vi "GetSetterAccessorInfo.vi"(8 "error in (no error)":errorcluster, 11 "PropertyBinder in":refnum<class "PropertyBinder.lvclass">) -> (0 "error out":errorcluster, 2 "SetterAccessorInfo":T1[](array[typedef]), 3 "PropertyBinder out":refnum<class "PropertyBinder.lvclass">)   [LabVIEW 2023, in "PropertyBinder.lvclass"]
uses:
  PropertyBinder.lvclass
  PropertyBinder.lvclass/PropertyBinder.ctl
  ClassReflector/AccessorTypeEnum.ctl
  ClassReflector/ClassReflector.lvclass
  ClassReflector/AccessorInfoCluster.ctl
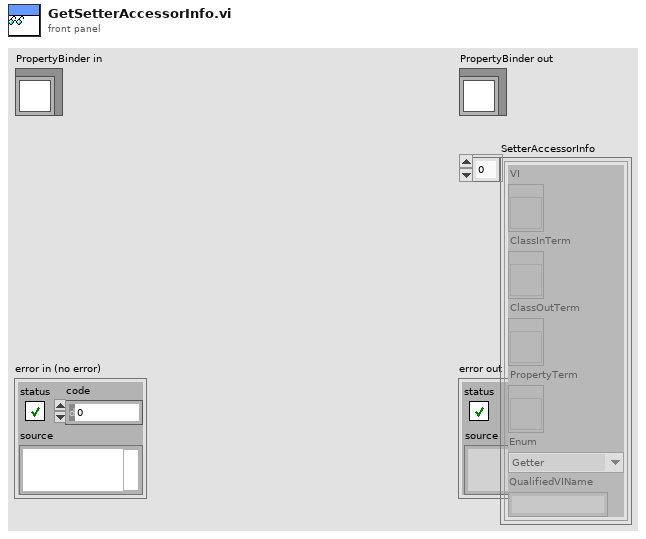
[diagram p1: front panel]
types:
  T1 = typedef "ClassReflector.lvclass/AccessorInfoCluster.ctl" = cluster{"VI":refnum<vi>, "ClassInTerm":refnum<vi>, "ClassOutTerm":refnum<vi>, "PropertyTerm":refnum<vi>, "Enum":T2, "QualifiedVIName":string}
  T2 = typedef "ClassReflector.lvclass/AccessorTypeEnum.ctl" = enum16{"Getter", "Setter"}
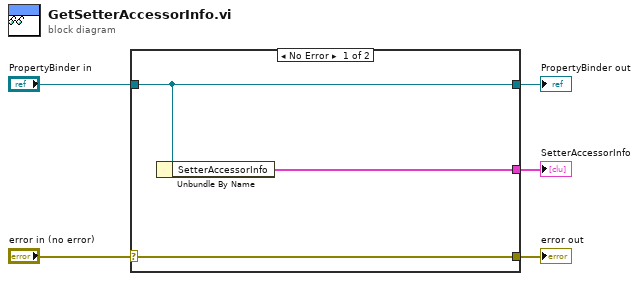
[diagram p0: block diagram]
diagram:
  n1 = case shown="No Error" "error in (no error)" {
    selector: "error in (no error)" -> [w8 w9]
    tunnel: [w8 w9] -> w4
    tunnel: [w7 w10] -> w2
    tunnel: "PropertyBinder in" -> [w7 w10]
    tunnel: [w6 _] -> w1
    frame No Error {
      n2 = Unbundle By Name(w7) -> ("SetterAccessorInfo"=w6:T1[])
    }
    frame Error {
    }
  }
  "error out" <- w4
  "PropertyBinder out" <- w2
  "SetterAccessorInfo" <- w1
